vi "Set Remote Terminal Address.vi"(8 "error in":errorcluster, 10 "terminal address":T1, 11 "remote terminal":T2 format="%.0x") -> (0 "error out":errorcluster, 3 "remote terminal out":T2 format="%.0x")   [LabVIEW 2020, in "AIM MIL-STD-1553 Scripting.lvlib"]
doc: "Sets the <b>terminal address</b> on the specified <b>remote terminal</b>."
uses:
  AIM MIL-STD-1553 Scripting.lvlib
  <vilib>/NI VeriStand/Custom Device API/Custom Device Item Ref.ctl
  Shared/Address.ctl
  Constants.vi
  <vilib>/NI VeriStand/Custom Device API/Set Item Property (U16).vi
  <vilib>/NI VeriStand/Custom Device API/Custom Device API.lvlib
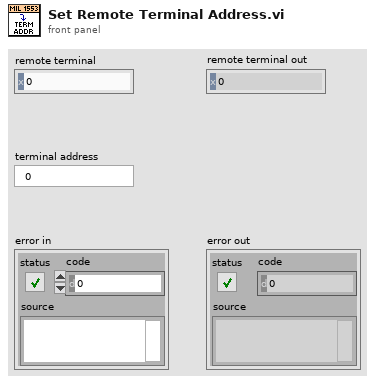
[diagram p1: front panel]
types:
  T1 = typedef "Address.ctl" = u16
  T2 = typedef "Custom Device API.lvlib/Custom Device Item Ref.ctl" = u64
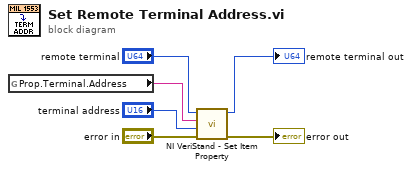
[diagram p0: block diagram]
diagram:
  n1 = global read "Constants.vi" "Prop.Terminal.Address"() -> (w1:string)
  n2 = call-poly <vilib>:"NI VeriStand - Set Item Property.vi"("error in (no error)"="error in", "Value"="terminal address", "Property Name"=w1, "Item Ref in"="remote terminal") -> ("error out"=→"error out":errorcluster, "Item Ref out"=→"remote terminal out":T2)  [unwired: 5 in, 1 out]
